vi "PH_OceanOpticsSpectrometer.set i Attr.vi"(0 "i ref in":refnum<vi>, 5 "error in (no error)":errorcluster) -> (14 "i ref out":refnum<vi>, 16 "i Attributes":T1={"GUI Refs"={"Delete"=refnum, "Spectrum"=refnum, "Display Width"=refnum, "Display Center"=refnum, "Save"=refnum, "Integration time"=refnum, "center wavelength"=refnum, "width"=refnum, "Wanted Trigger Mode"=refnum, "Current Trigger Mode"=refnum, "Trigger Info"=refnum, "Model"=refnum, "Driver"=refnum, "Firmware"=refnum}, "Display"={"Width"=50.0, "Center"=1054.0}, "VISA resource name"="N/A", "Integration time [ms]"={"Current Value"=100, "Wanted Value"=100}, "Trigger"={"Current value"=enum."Normal", "Wanted value"=enum."Normal"}, "Default VISA Timeout"=0, "Last Data"={"Wavelength Bins"=[], "Spectrum by Pixels"=[]}} {"Integration time [ms]"."Wanted Value" min=1 max=500 step=1; "Integration time [ms]"."Current Value" min=1 max=500 step=1}, 19 "error out":errorcluster)   [LabVIEW 2014, in "PH_OceanOpticsSpectrometer.lvlib"]
doc: "This VI reads information from the database and writes it to own attributes."
uses:
  PH_OceanOpticsSpectrometer.lvlib
  PH_OceanOpticsSpectrometer.i attribute.ctl
  PH_OceanOpticsSpectrometer.Trigger.ctl
  PH_Basics/PH_Common/PH_Common.lvlib
  CS_Core/CSSystem/CSSystemLib/CSSystemLib.lvlib
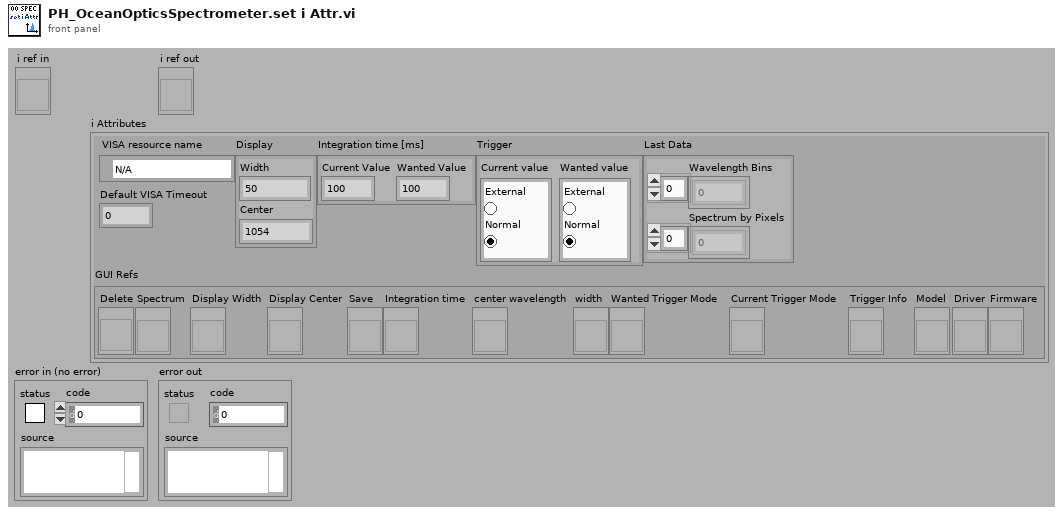
[diagram p1: front panel]
types:
  T1 = typedef "PH_OceanOpticsSpectrometer.lvlib/PH_OceanOpticsSpectrometer.i attribute.ctl" = cluster{"GUI Refs":cluster{"Delete":refnum<vi>, "Spectrum":refnum<vi>, "Display Width":refnum<vi>, "Display Center":refnum<vi>, "Save":refnum<vi>, "Integration time":refnum<vi>, "center wavelength":refnum<vi>, "width":refnum<vi>, "Wanted Trigger Mode":refnum<vi>, "Current Trigger Mode":refnum<vi>, "Trigger Info":refnum<vi>, "Model":refnum<vi>, "Driver":refnum<vi>, "Firmware":refnum<vi>}, "Display":cluster{"Width":dbl, "Center":dbl}, "VISA resource name":refnum<visa-resource-name>, "Integration time [ms]":cluster{"Current Value":u16, "Wanted Value":u16}, "Trigger":cluster{"Current value":T2, "Wanted value":T2}, "Default VISA Timeout":u32, "Last Data":cluster{"Wavelength Bins":dbl[], "Spectrum by Pixels":dbl[]}}
  T2 = typedef "PH_OceanOpticsSpectrometer.lvlib/PH_OceanOpticsSpectrometer.Trigger.ctl" = enum32{"External", "Normal"}
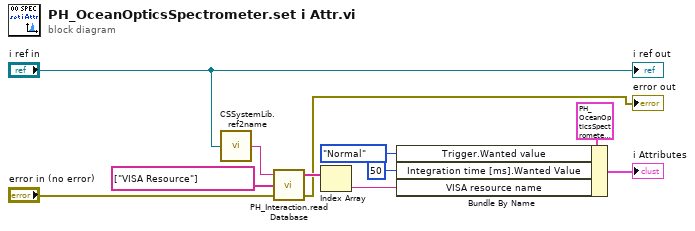
[diagram p0: block diagram]
diagram:
  n1 = call "CSSystemLib.ref2name.vi"("obj refnum"="i ref in") -> ("name"=w6:string)
  n2 = call "PH_Interaction.read Database.vi"("error in (no error)"="error in (no error)", "Strings to search for"=string[] ["VISA Resource"], "DB Entry to read"=w6) -> ("error out"=→"error out":errorcluster, "Values"=w9:string[])  [unwired: 1 in]
  n3 = Index Array(array=w9) -> (element=w8:string)  [unwired: 1 in]
  n4 = Bundle By Name(cluster=T1 {"GUI Refs"={"Delete"=refnum, "Spectrum"=refnum, "Display Width"=refnum, "Display Center"=refnum, "Save"=refnum, "Integration time"=refnum, "center wavelength"=refnum, "width"=refnum, "Wanted Trigger Mode"=refnum, "Current Trigger Mode"=refnum, "Trigger Info"=refnum, "Model"=refnum, "Driver"=refnum, "Firmware"=refnum}, "Display"={"Width"=0.0, "Center"=0.0}, "VISA resource name"="", "Integration time [ms]"={"Current Value"=0, "Wanted Value"=0}, "Trigger"={"Current value"=enum."External", "Wanted value"=enum."External"}, "Default VISA Timeout"=0, "Last Data"={"Wavelength Bins"=[], "Spectrum by Pixels"=[]}} ("i attribute"), "Trigger.Wanted value"=PH_OceanOpticsSpectrometer.Trigger."Normal", "Integration time [ms].Wanted Value"=u16 50 ("y"), "VISA resource name"=w8) -> (→"i Attributes":T1)
  "i ref out" <- "i ref in"
